vi "ErrorRun.vi"(8 "error in (no error)":errorcluster) -> (0 "error out":errorcluster)   [LabVIEW 2017, in "ErrorMonitor.lvlib"]
uses:
  ErrorMonitor.lvlib
  UEFGV/Type Def/UEFGV_States.ctl
  TypeDefs/LoopStates.ctl
  Queue/TypeDefs/queueFGVState.ctl
  loggingModule/loggingModule.lvlib
  programControl/programControl.lvlib
panel:
  out "Shutdown":bool
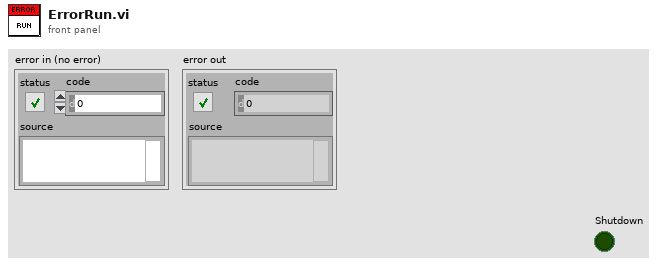
[diagram p1: front panel]
types:
  T1 = typedef "UEFGV_States.ctl" = enum16{"Create", "Get", "Destroy"}
  T2 = typedef "LoopStates.ctl" = enum16{"start", "wait", "run", "end"}
  T3 = typedef "ErrorMonitor.lvlib/queueFGVState.ctl" = enum16{"obtain", "enqueue low priority", "enqueue high priority", "dequeue", "release"}
  T4 = typedef "ErrorMonitor.lvlib/message.ctl" = cluster{"calling module":string, "message":string, "Data":variant}
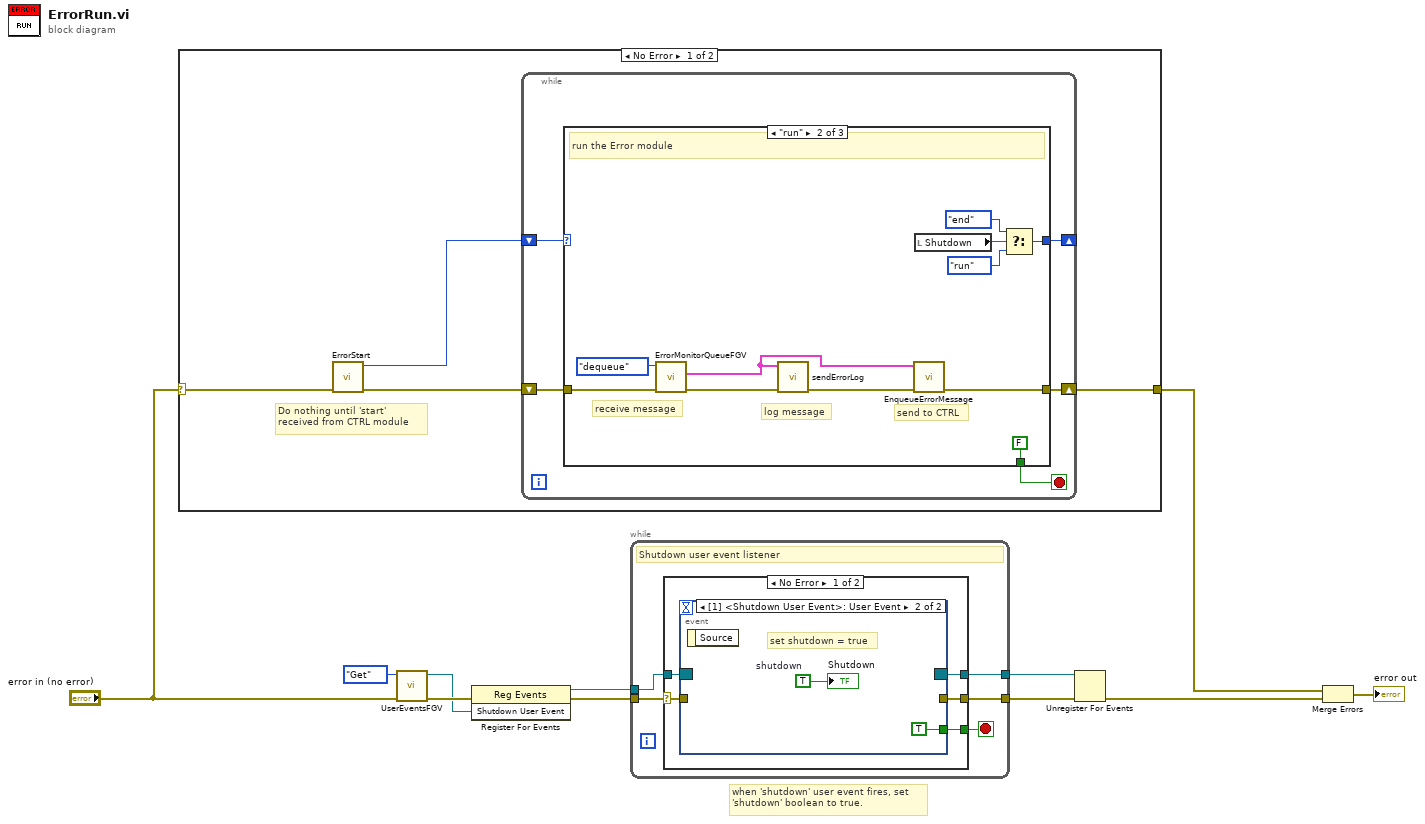
[diagram p0: block diagram]
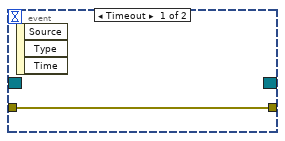
[diagram p2: hidden frame]
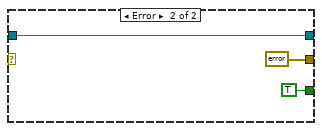
[diagram p3: hidden frame]
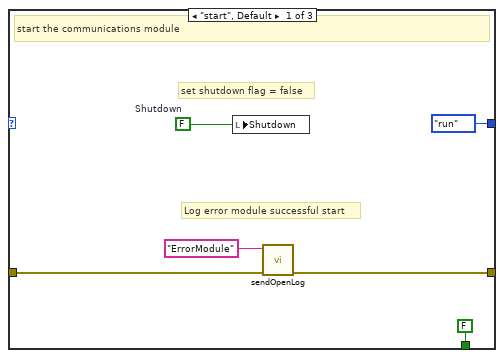
[diagram p4: hidden frame]
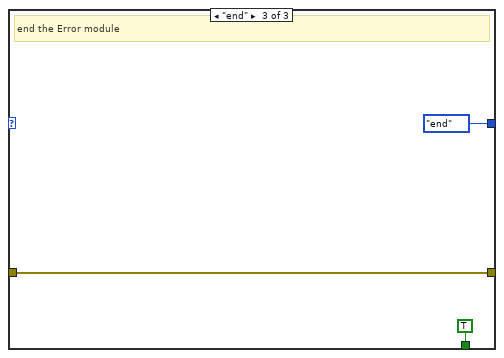
[diagram p5: hidden frame]
diagram:
  # "when 'shutdown' user event fires, set\n'shutdown' boolean to true."
  n1 = case shown="No Error" "error in (no error)" {
    selector: "error in (no error)" -> [w15 w41]
    tunnel: [w12 w41] -> w5
    frame No Error {
      # "Do nothing until 'start'\nreceived from CTRL module"
      n2 = call "ErrorStart.vi"("error in (no error)"=w15) -> ("error out"=w13:errorcluster, "message out"=w14:T2)  [unwired: 9 in]
      n3 = while {
        shift-right: [w16] -> _
        shift-left: w14 -> [w20]
        shift-right: [w17] -> w12
        shift-left: w13 -> [w18]
        stop <- w19 stop-if-true
        n4 = case shown="\"run\"" w20 {
          tunnel: [FALSE FALSE TRUE] -> w19
          tunnel: w18 -> [w23 w32 w39]
          tunnel: [w22 w28 w39] -> w17
          tunnel: [LoopStates."run" ("message out") w33 LoopStates."end" ("message out")] -> w16
          frame "start", Default {
            w25 = FALSE  # Shutdown
            # "Log error module successful start"
            # "set shutdown flag = false"
            # "start the communications module"
            n5 = local write "Shutdown"(w25) -> ()
            n6 = call "sendOpenLog.vi"("error in (no error)"=w23, "source"="ErrorModule") -> ("error out"=w22:errorcluster)  [unwired: 9 in]
          }
          frame "run" {
            # "send to CTRL"
            # "receive message"
            # "log message"
            # "run the Error module"
            n7 = call "ErrorMonitorQueueFGV.vi"("error in (no error)"=w32, "Enum"=queueFGVState."dequeue") -> ("error out"=w30:errorcluster, "message out"=w27:T4)  [unwired: 8 in]
            n8 = call "sendErrorLog.vi"("error in (no error)"=w30, "message out"=w27) -> ("error out"=w29:errorcluster)  [unwired: 9 in]
            n9 = call "EnqueueErrorMessage.vi"("error in (no error)"=w29, "message out"=w27) -> ("error out"=w28:errorcluster)  [unwired: 9 in]
            n10 = local read "Shutdown"() -> (w36:bool)
            n11 = Select(t=LoopStates."end" ("message out"), s=w36, f=LoopStates."run" ("message out")) -> (s? t:f=w33:T2)
          }
          frame "end" {
            # "end the Error module"
          }
        }
      }
    }
    frame Error {
    }
  }
  n12 = call "UserEventsFGV.vi"("error in (no error)"="error in (no error)", "Command"=UEFGV_States."Get") -> ("error out"=w9:errorcluster, "Shutdown User Event"=w8:refnum<user-event>)  [unwired: 8 in]
  n13 = register-events(error in=w9, w8) -> (reference out=w11:refnum<event-registration>, error out=w6:errorcluster)  [unwired: 1 in]
  n14 = while {
    tunnel: w11 -> [w46]
    tunnel: [w45] -> w10
    tunnel: w6 -> [w43]
    tunnel: [w42] -> w7
    stop <- w44 stop-if-true
    # "Shutdown user event listener"
    n15 = case shown="No Error" w43 {
      selector: w43 -> [w48 _]
      tunnel: w46 -> [w51 w56]
      tunnel: [w50 w56] -> w45
      tunnel: [w49 TRUE] -> w44
      tunnel: [w47 errorcluster {"status"=FALSE, "code"=0, "source"=""} ("error out")] -> w42
      frame No Error {
        n16 = event shown="[1] <Shutdown User Event>: User Event" {
          selector: w51 -> [_ _]
          dyn-events: [_ _] -> w50
          timeout: _ -> [_ _]
          tunnel: w48 -> [w52 _]
          tunnel: [w52 _] -> w47
          tunnel: [_ TRUE] -> w49
          event Timeout {
            n17 = event-data() -> ()  [unwired: 1 in, 3 out]
          }
          event User Event {
            w53 = TRUE  # shutdown
            # "set shutdown = true"
            n18 = event-data() -> ()  [unwired: 1 in, 1 out]
            "Shutdown" <- w53
          }
        }
      }
      frame Error {
      }
    }
  }
  n19 = Unregister For Events(event registration refnum=w10, error in=w7) -> (error out=w4:errorcluster)
  n20 = Merge Errors(w5, w4) -> (→"error out":errorcluster)
